vi "UpdateCamera.vi"(8 "error in (no error)":errorcluster, 11 "Render Window in":refnum<class "Render Window.lvclass">) -> (0 "error out":errorcluster, 3 "Render Window out":refnum<class "Render Window.lvclass">)   [LabVIEW 2015, in "Render Window.lvclass"]
uses:
  Render Window.lvclass
  Render Window.lvclass/Render Window.ctl
  3D Scene/3D Scene.lvclass
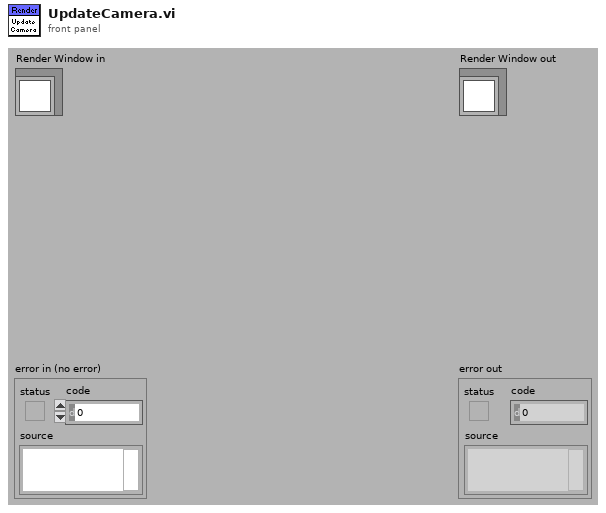
[diagram p1: front panel]
types:
  T1 = typedef "3D Point.ctl" = cluster{"X":sgl, "Y":sgl, "Z":sgl}
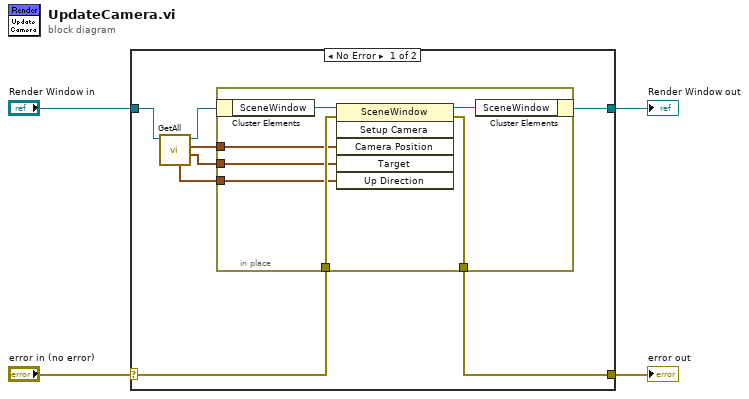
[diagram p0: block diagram]
diagram:
  n1 = case shown="No Error" "error in (no error)" {
    selector: "error in (no error)" -> [w12 w21]
    tunnel: [w11 w21] -> w3
    tunnel: [w10 w20] -> w1
    tunnel: "Render Window in" -> [w9 w20]
    frame No Error {
      n2 = call "GetAll.vi"("3D Scene in"=w9) -> ("Target"=w6:T1, "Position"=w7:T1, "3D Scene out"=w8:refnum<class "Render Window.lvclass">, "Up"=w5:T1)  [unwired: 6 in, 1 out]
      n3 = in-place {
        in-place-border: w12 -> [w18]
        in-place-border: [w17] -> w11
        in-place-border: w7 -> [w15]
        in-place-border: w6 -> [w14]
        in-place-border: w5 -> [w13]
        n4 = in-place-cluster #1(w8) -> ("SceneWindow"=w16:refnum<vi>)
        n5 = invoke class="SceneWindow" method="Setup Camera"(reference=w16, error in=w18, "Camera Position"=w15, "Target"=w14, "Up Direction"=w13) -> (reference out=w19:refnum<vi>, error out=w17:errorcluster)  [unwired: 1 in, 4 out]
        n6 = in-place-cluster #1("SceneWindow"=w19) -> (w10:refnum<class "Render Window.lvclass">)
      }
    }
    frame Error {
    }
  }
  "error out" <- w3
  "Render Window out" <- w1
